vi "Operation UI.vi"(0 "A":dbl, 5 "B":dbl, 7 "Calculate":bool, 9 "DVR In":refnum<data-value>, 11 "Error In":errorcluster, 12 "Stop":refnum<user-event>, 13 "Class Data":refnum<user-event>) -> (4 "C":dbl, 10 "DVR Out":refnum<data-value>, 15 "Error out":errorcluster)   [LabVIEW 2023, in "Multiply.lvclass"]
doc: "The VI contains the addition operation UI that accepts two input numbers and performs multiplication operation and displays the output when user clicks calculate button"
uses:
  Multiply.lvclass
  Arithemtic Operation/Arithemetic Operation.lvclass
  Typedef/User Event Operations.ctl
panel:
  # "MULTIPLICATION"
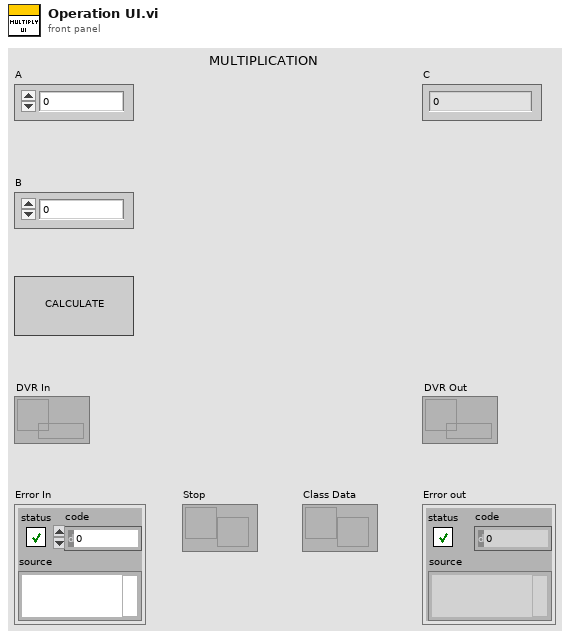
[diagram p1: front panel]
types:
  T1 = typedef "User Event Operations.ctl" = enum16{"Obtain", "Generate", "Release"}
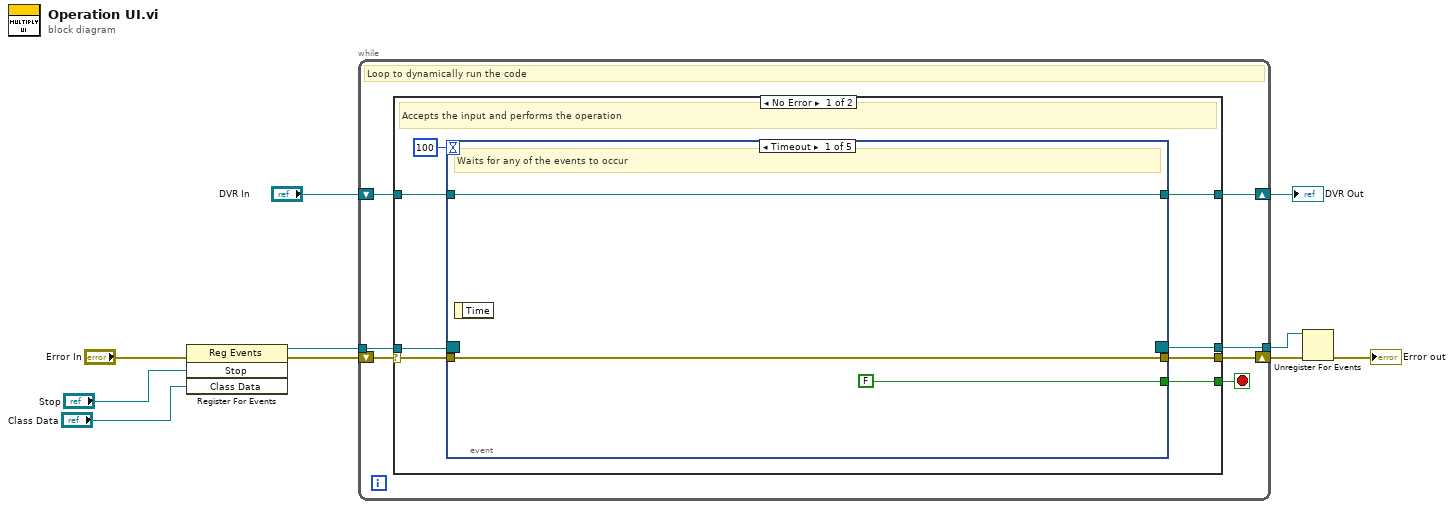
[diagram p0: block diagram]
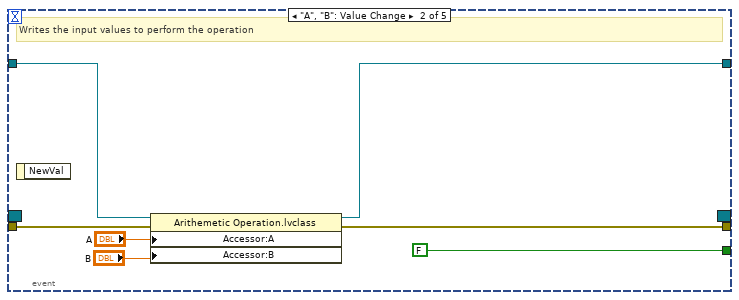
[diagram p2: hidden frame]
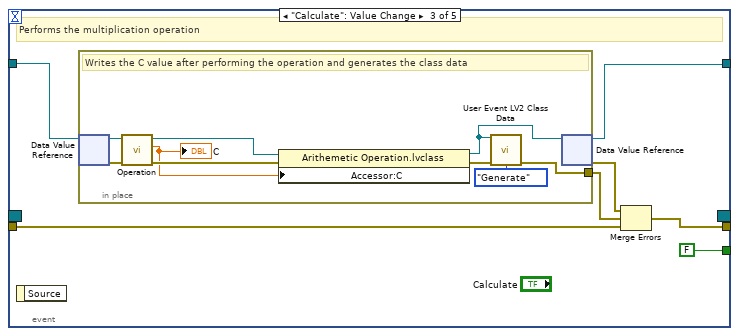
[diagram p3: hidden frame]
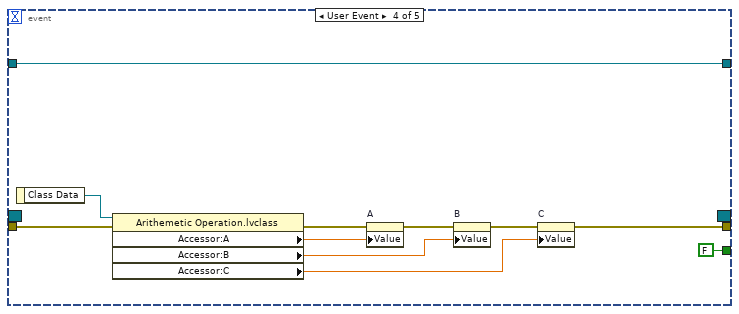
[diagram p4: hidden frame]
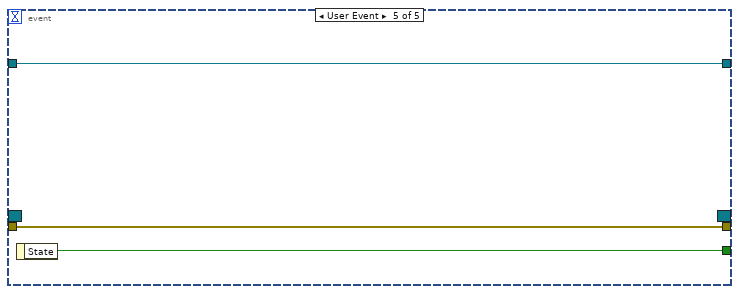
[diagram p5: hidden frame]
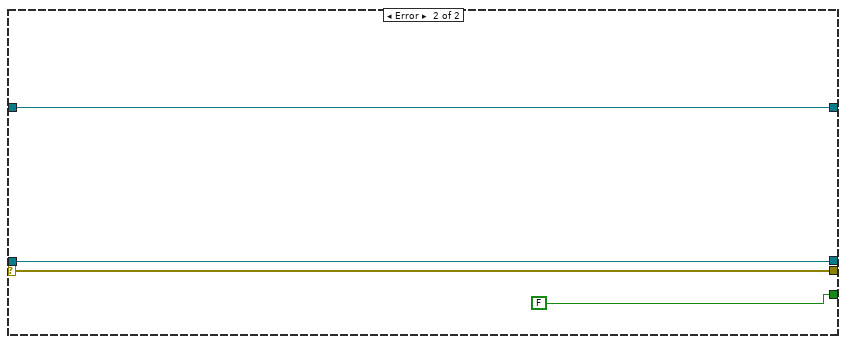
[diagram p6: hidden frame]
diagram:
  n1 = register-events(error in="Error In", "Stop", "Class Data") -> (reference out=w7:refnum<event-registration>, error out=w8:errorcluster)  [unwired: 1 in]
  n2 = while {
    shift-right: [w16] -> w10
    shift-left: w8 -> [w17]
    shift-right: [w14] -> w3
    shift-left: "DVR In" -> [w15]
    tunnel: w7 -> [w13]
    tunnel: [w12] -> w5
    stop <- w11 stop-if-true
    # "Loop to dynamically run the code"
    n3 = case shown="No Error" w17 {
      selector: w17 -> [w23 w69]
      tunnel: [w22 w69] -> w16
      tunnel: [w24 w68] -> w14
      tunnel: w15 -> [w25 w68]
      tunnel: w13 -> [w20 w67]
      tunnel: [w19 w67] -> w12
      tunnel: [w18 FALSE] -> w11
      frame No Error {
        # "Accepts the input and performs the operation"
        n4 = event shown="[0] Timeout" {
          selector: w20 -> [_ _ _ _ _]
          dyn-events: [_ _ _ _ _] -> w19
          timeout: 100 -> [_ _ _ _ _]
          tunnel: [w28 w30 w40 w62 w64] -> w24
          tunnel: w25 -> [w28 w33 w41 w62 w64]
          tunnel: w23 -> [w27 w35 w39 w61 w65]
          tunnel: [w27 w34 w38 w56 w65] -> w22
          tunnel: [FALSE FALSE FALSE FALSE ("State") w63] -> w18
          event Timeout {
            # "Waits for any of the events to occur"
            n5 = event-data() -> ()  [unwired: 1 in, 1 out]
          }
          event "A", "B": Value Change {
            # "Writes the input values to perform the operation"
            n6 = event-data() -> ()  [unwired: 1 in, 1 out]
            n7 = property class="Arithemetic Operation.lvclass"(reference=w33, error in=w35, "Accessor:A"="A", "Accessor:B"="B") -> (reference out=w30:refnum<data-value>, error out=w34:errorcluster)
          }
          event "Calculate": Value Change {
            # "Performs the multiplication operation"
            n8 = event-data() -> ()  [unwired: 1 in, 1 out]
            n9 = in-place {
              in-place-border: [w43] -> w36
              # "Writes the C value after performing the operation and generates the class data"
              n10 = in-place-dvr #1(w41) -> (w45:refnum<class "Arithemetic Operation.lvclass">, w46:errorcluster)
              n11 = call-dynamic "Operation.vi"("Error In"=w46, "Arithemetic Operation in"=w45) -> ("Error Out"=w51:errorcluster, "C"=w48:dbl, "Arithemetic Operation out"=w49:refnum<class "Arithemetic Operation.lvclass">)  [unwired: 7 in]
              "C" <- w48
              n12 = property class="Arithemetic Operation.lvclass"(reference=w49, error in=w51, "Accessor:C"=w48) -> (reference out=w44:refnum<class "Arithemetic Operation.lvclass">, error out=w50:errorcluster)
              n13 = call "User Event LV2 Class Data.vi"("Class Data"=w44, "Error In"=w50, "Operation"=User_Event_Operations."Generate") -> ("Error Out"=w43:errorcluster)  [unwired: 11 in, 1 out]
              n14 = in-place-dvr #1(w44) -> (w40:refnum<data-value>, w37:errorcluster)
            }
            n15 = Merge Errors(w37, w36, w39) -> (w38:errorcluster)
          }
          event User Event {
            n16 = event-data() -> ("Class Data"=w59:refnum<class "Arithemetic Operation.lvclass">)  [unwired: 1 in]
            n17 = property class="Arithemetic Operation.lvclass"(reference=w59, error in=w61) -> (error out=w60:errorcluster, "Accessor:A"=w55:dbl, "Accessor:B"=w54:dbl, "Accessor:C"=w53:dbl)  [unwired: 1 out]
            n18 = property on="A" class="DigNum (strict)"(error in=w60, "Value"=w55) -> (error out=w58:errorcluster)  [unwired: 1 in, 1 out]
            n19 = property on="B" class="DigNum (strict)"(error in=w58, "Value"=w54) -> (error out=w57:errorcluster)  [unwired: 1 in, 1 out]
            n20 = property on="C" class="DigNum (strict)"(error in=w57, "Value"=w53) -> (error out=w56:errorcluster)  [unwired: 1 in, 1 out]
          }
          event User Event {
            n21 = event-data() -> ("State"=w63:bool)  [unwired: 1 in]
          }
        }
      }
      frame Error {
      }
    }
  }
  "DVR Out" <- w3
  n22 = Unregister For Events(event registration refnum=w5, error in=w10) -> (error out=→"Error out":errorcluster)
